vi "Generate load Current Sequence.vi"(0 "Load SMU Reference":refnum<k15>, 5 "sequence name":string="CurrentSequence", 7 "Total Aquisition Time (s)":dbl format="%#_13g", 9 "Load Current Sequence":dbl[](array[numeric]), 11 "error in (no error)":errorcluster) -> (4 "SMU Reference":refnum<k15>, 15 "error out":errorcluster)   [LabVIEW 2020, in "LDO Load Transient.lvlib"]
uses:
  LDO Load Transient.lvlib
  <instrlib>/niDCPower/nidcpower.llb/niDCPower Wait For Event - Event.ctl
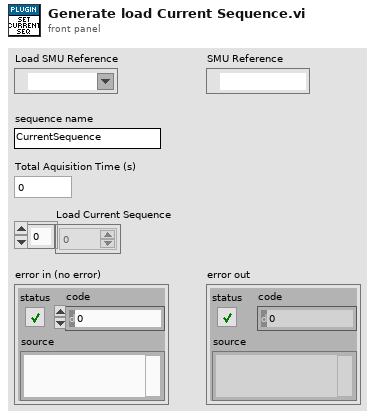
[diagram p1: front panel]
types:
  T1 = typedef "niDCPower Wait For Event - Event.ctl" = i32
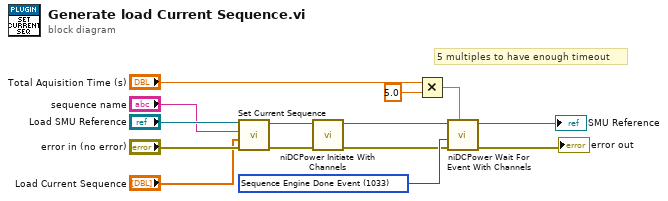
[diagram p0: block diagram]
diagram:
  w14 = T1 1033 items=["Source Complete Event"=1030, "Measure Complete Event"=1031, "Sequence Iteration Complete Event"=1032, "Sequence Engine Done Event"=1033] ("event")
  # "5 multiples to have enough timeout"
  n1 = call "Set Current Sequence.vi"("error in (no error)"="error in (no error)", "Load Current Sequence"="Load Current Sequence", "Sequence Name"="sequence name", "Load SMU Reference"="Load SMU Reference") -> ("error out"=w7:errorcluster, "Load SMU Reference"=w5:refnum<k15>)  [unwired: 6 in]
  n2 = call <instrlib>:"niDCPower Initiate With Channels.vi"("error in (no error)"=w7, "instrument handle"=w5) -> ("error out"=w13:errorcluster, "instrument handle out"=w12:refnum<k15>)  [unwired: 8 in]
  n3 = Multiply(x="Total Aquisition Time (s)", y=5.0 ("value")) -> (x*y=w11:dbl)
  n4 = call <instrlib>:"niDCPower Wait For Event With Channels.vi"("timeout (sec)"=w11, "error in (no error)"=w13, "event"=w14, "instrument handle"=w12) -> ("error out"=→"error out":errorcluster, "instrument handle out"=→"SMU Reference":refnum<k15>)  [unwired: 6 in]
